vi "ADCCalc.vi"(1 "Rsense":dbl, 2 "Gain":dbl, 3 "DATA":u16) -> (0 "NumOut":dbl)   [LabVIEW 2017]
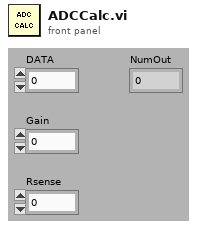
[diagram p1: front panel]
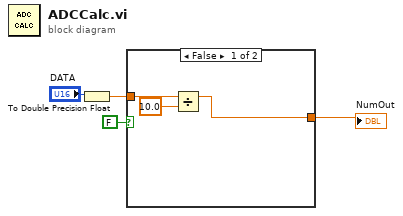
[diagram p0: block diagram]
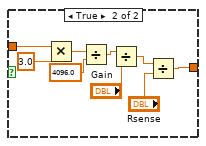
[diagram p2: hidden frame]
diagram:
  n1 = To Double Precision Float(number="DATA") -> (double precision float=w3:dbl)
  n2 = case shown="False" FALSE {
    tunnel: [w6 w16] -> w4
    tunnel: w3 -> [w7 w8]
    frame False {
      n3 = Divide(x=w7, y=10.0) -> (x/y=w6:dbl)
    }
    frame True {
      n4 = Multiply(x=w8, y=3.0) -> (x*y=w10:dbl)
      n5 = Divide(x=w10, y=4096.0) -> (x/y=w12:dbl)
      n6 = Divide(x=w12, y="Gain") -> (x/y=w14:dbl)
      n7 = Divide(x=w14, y="Rsense") -> (x/y=w16:dbl)
    }
  }
  "NumOut" <- w4
